vi "ListenForSubscriber.vi"(2 "LogPath in":path, 3 "ROS":T1) -> (0 "heard?":errorcluster, 1 "server":refnum<k5>)   [LabVIEW 2016]
doc: "Listens on the TCP network for a subscriber"
uses:
  _ROSControl.ctl
  _ROSDirection.ctl
  Console/Servers/ServerSubs/MyState.ctl
  _ROSDefinition.vi
panel:
  out "LogPath out":path
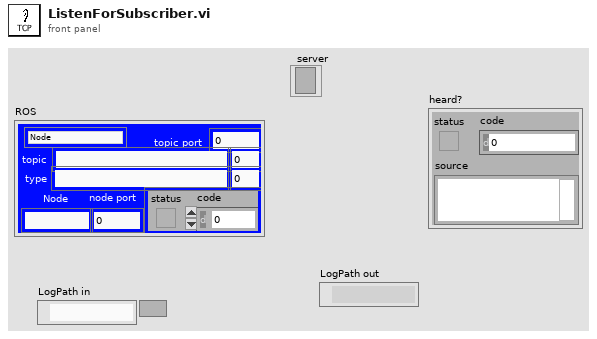
[diagram p1: front panel]
types:
  T1 = typedef "_ROSControl.ctl" = cluster{"topic port":u16, "Node":string, "topic":string, "type":string, "node port":u16, "error ":errorcluster, "Direction":T2, "Update (ms)":u16, "FIFO size":u16}
  T2 = typedef "_ROSDirection.ctl" = enum16{"Node", "Publisher", "Subscriber", "ServiceClient", "ServiceProvider"}
  T3 = typedef "MyState.ctl" = enum16{"No Connection", "Registered", "Connected", "Close"}
  T4 = typedef "ROSLog.ctl" = cluster{"Sent":string, "Reply":string, "MethodName":string, "success":bool, "Dir1":string, "Dir2":string, "Time Stamp":string, "error":errorcluster, "Preamble":string, "Midamble":string, "Postamble":string}
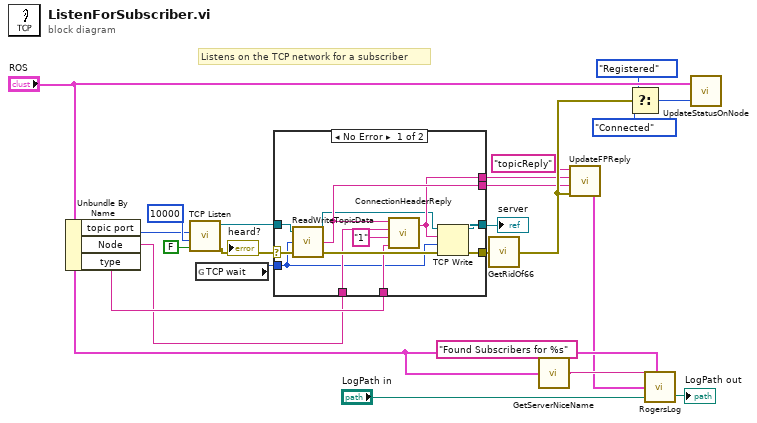
[diagram p0: block diagram]
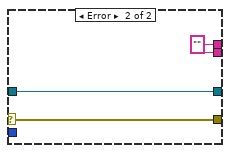
[diagram p2: hidden frame]
diagram:
  # "Listens on the TCP network for a subscriber"
  n1 = Unbundle By Name("ROS") -> ("topic port"=w4:u16, "Node"=w5:string, "type"=w6:string)
  n2 = call "TCP Listen.vi"("resolve remote address (T)"=FALSE, "timeout ms (wait forever: -1)"=10000, "port"=w4) -> ("error out"=w1:errorcluster, "connection ID"=w2:refnum<k5>)  [unwired: 4 in, 3 out]
  "heard?" <- w1
  n3 = global read "_ROSDefinition.vi" "TCP wait"() -> (w7:i32)
  n4 = case shown="No Error" w1 {
    selector: w1 -> [w25 w38]
    tunnel: [w35 w38] -> w13
    tunnel: [w34 w37] -> w12
    tunnel: [w33 w36] -> w10
    tunnel: [w32 w36] -> w9
    tunnel: w7 -> [w24 _]
    tunnel: w6 -> [w28 _]
    tunnel: w5 -> [w27 _]
    tunnel: w2 -> [w26 w37]
    frame No Error {
      n5 = call "ReadWriteTopicData.vi"("error in (no error)"=w25, "timeout ms (1000)"=w24, "connection ID in"=w26) -> ("error out"=w31:errorcluster, "data out"=w33:string, "connection ID out"=w30:refnum<k5>)
      n6 = call "ConnectionHeaderReply.vi"("type"=w28, "Latching"="1", "Caller ID"=w27, "TCPROS Connection Header"=w33) -> ("Connection Response"=w32:string)  [unwired: 1 in]
      n7 = TCP Write(connection ID=w30, data in=w32, error in (no error)=w31, 9:w24) -> (connection ID out=w34:refnum<k5>, error out=w35:errorcluster)  [unwired: 1 out]
    }
    frame Error {
      w36 = "" ("Connection Response")
    }
  }
  "server" <- w12
  n8 = call "GetRidOf66.vi"("error in (no error)"=w13) -> ("error out"=w15:errorcluster)
  n9 = call "GetServerNiceName.vi"("ROS"="ROS", "Text to add"="Found Subscribers for %s") -> ("String"=w20:string)
  n10 = call "UpdateFPReply.vi"("error in (no error)"=w15, "Reply"=w10, "Sent"=w9, "method"="topicReply") -> ("Log"=w17:T4)
  n11 = Select(t=MyState."Registered" ("MyState"), s=w15, f=MyState."Connected" ("MyState")) -> (s? t:f=w22:T3)
  n12 = call "RogersLog.vi"("Text to add"=w20, "ROS"="ROS", "Log"=w17, "LogPath in"="LogPath in") -> ("LogPath out"=→"LogPath out":path)  [unwired: 1 in, 1 out]
  n13 = call "UpdateStatusOnNode.vi"("MyState"=w22, "ROS"="ROS") -> ()  [unwired: 1 in, 1 out]
